vi "Apply Exclusion Value.vi"(7 "Excluded?":bool, 10 "Filtered value in":bool) -> (2 "Final Filtered Value":bool)   [LabVIEW 2016, in "Assert API Components.lvlib" / "Base Filter.lvclass"]
doc: "Takes in the status of the current filter, and then either excludes or includes the value depending on what has been set on excluded"
uses:
  Base Filter.lvclass
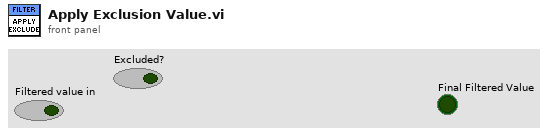
[diagram p1: front panel]
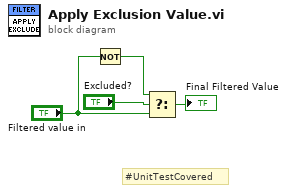
[diagram p0: block diagram]
diagram:
  # "#UnitTestCovered"
  n1 = Not(x="Filtered value in") -> (.not. x?=w4:bool)
  n2 = Select(t=w4, s="Excluded?", f="Filtered value in") -> (s? t:f=→"Final Filtered Value":bool)
